vi "Database-GetDBsets.vi"(7 "Idx":i32, 10 "Variant":string) -> (0 "Found":bool, 1 "Variant Sets":T2, 2 "Variant Idx":T1, 3 "Sets":T3, 4 "PrevVariantsInUse":string[](array[string]))   [LabVIEW 2016]
uses:
  Database.Global.vi
  Database.Data.Sets.ctl
  Database.Data.Variant.Sets.ctl
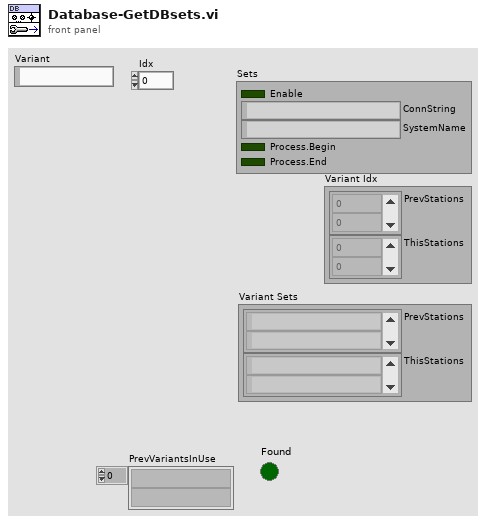
[diagram p1: front panel]
types:
  T1 = cluster{"PrevStations":i32[], "ThisStations":i32[]}
  T2 = typedef "Database.Data.Variant.Sets.ctl" = cluster{"PrevStations":string[], "ThisStations":string[]}
  T3 = typedef "Database.Data.Sets.ctl" = cluster{"Enable":bool, "ConnString":string, "SystemName":string, "Process.Begin":bool, "Process.End":bool}
  T4 = typedef "Cache.Status.Fglb.Data.ctl" = cluster{"Changeover":string, "CheckStatus":T5, "NewData":T6}
  T5 = typedef "PLC.DataBlock.PCcheckstatus.ctl" = cluster{"Ref":string, "Serial":string, "StatusPrev":i8, "StatusThis":i8, "Repetitions":u8}
  T6 = typedef "PLC.DataBlock.PLCvalues.ctl" = cluster{"Status":u8, "Ref1":string, "Serial1":string, "Ref2":string, "Serial2":string, "Values":sgl[]}
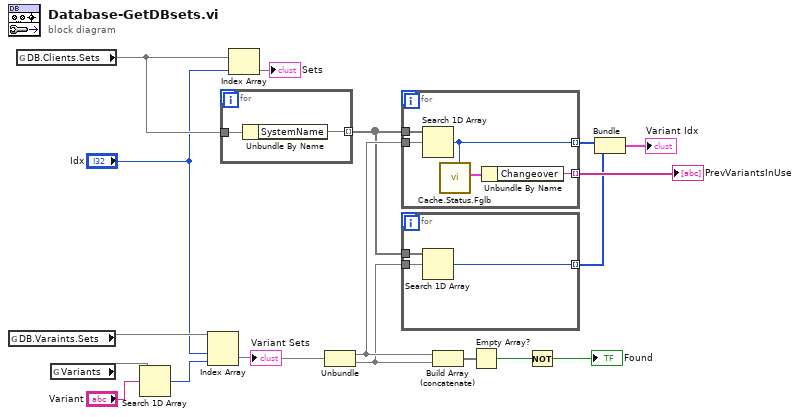
[diagram p0: block diagram]
diagram:
  n1 = global read "Database.Global.vi" "DB.Varaints.Sets"() -> (w18)
  n2 = global read "Database.Global.vi" "DB.Clients.Sets"() -> (w9)
  n3 = global read "Database.Global.vi" "Variants"() -> (w17)
  n4 = Search 1D Array(1D array=w17, element="Variant") -> (index of element=w14:i32)  [unwired: 1 in]
  n5 = Index Array(array=w18, index (row)="Idx", index (col)=w14) -> (element=w13)
  "Variant Sets" <- w13
  n6 = for {
    tunnel: w9 -> [w20]
    tunnel: [w19] -> w5 mode=indexing
    n7 = Unbundle By Name(w20) -> ("SystemName"=w19)
  }
  n8 = Index Array(array=w9, index="Idx") -> (element=→"Sets")
  n9 = Unbundle(w13) -> (w8, w4)
  n10 = for {
    tunnel: w5 -> [w25]
    tunnel: w8 -> [w24]
    tunnel: [w22] -> w7 mode=indexing
    tunnel: [w21] -> w3 mode=indexing
    n11 = Search 1D Array(1D array=w25, element=w24) -> (index of element=w21:i32)  [unwired: 1 in]
    n12 = call "Cache.Status.Fglb.vi"("SystemIdx"=w21) -> ("Data"=w23:T4)  [unwired: 9 in, 1 out]
    n13 = Unbundle By Name(w23) -> ("Changeover"=w22:string)
  }
  "PrevVariantsInUse" <- w7
  n14 = for {
    tunnel: w5 -> [w28]
    tunnel: w4 -> [w27]
    tunnel: [w26] -> w2 mode=indexing
    n15 = Search 1D Array(1D array=w28, element=w27) -> (index of element=w26:i32)  [unwired: 1 in]
  }
  n16 = Build Array (concatenate)(w8, w4) -> (w12:void[])
  n17 = Empty Array?(array=w12) -> (empty?=w11:bool)
  n18 = Not(x=w11) -> (.not. x?=→"Found":bool)
  n19 = Bundle(w3, w2) -> (→"Variant Idx":cluster{i32[], i32[]})  [unwired: 1 in]
